vi "ble_search_characteristic_declaration_handle.vi"(8 "error in (no error)":errorcluster, 9 "Characteristic UUID":string, 10 "Service UUID":string, 11 "Handle table":string[][](array[string])) -> (0 "error out":errorcluster, 2 "Handle":string)   [LabVIEW 2013]
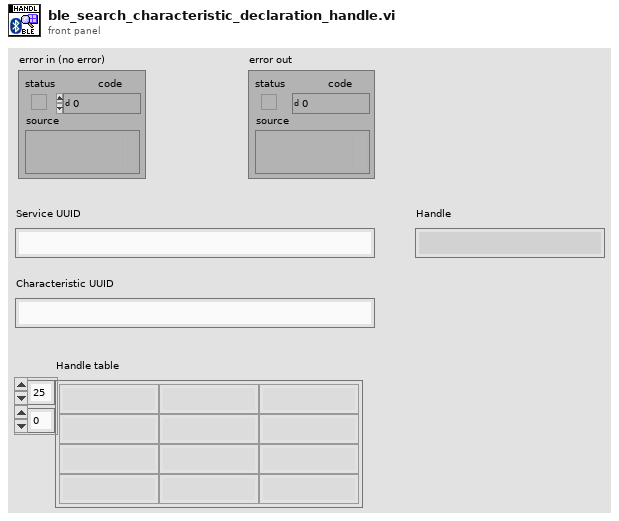
[diagram p1: front panel]
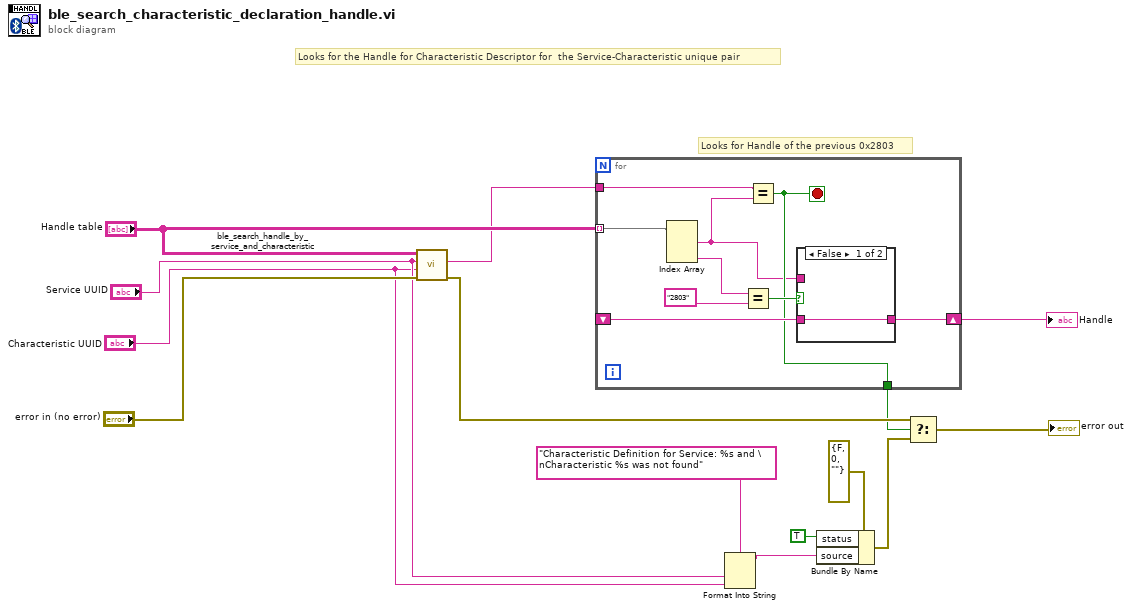
[diagram p0: block diagram]
diagram:
  # "Looks for Handle of the previous 0x2803"
  # "Looks for the Handle for Characteristic Descriptor for  the Service-Characteristic unique pair"
  n1 = call "ble_search_handle_by_service_and_characteristic.vi"("error in (no error)"="error in (no error)", "Characteristic UUID"="Characteristic UUID", "Service UUID"="Service UUID", "Handle table"="Handle table") -> ("error out"=w8:errorcluster, "Handle"=w6:string)  [unwired: 6 in]
  n2 = for {
    tunnel: "Handle table" -> [w23] mode=indexing
    tunnel: w6 -> [w22]
    shift-right: [w19] -> w3
    shift-left: _ -> [w18]
    tunnel: [w17] -> w5
    stop <- w17 stop-if-true
    n3 = Index Array(array=w23) -> (element #1=w16:string, element #3=w15:string)  [unwired: 3 in, 1 out]
    n4 = Equal?(x=w15, y="2803") -> (x = y?=w20:bool)
    n5 = Equal?(x=w22, y=w16) -> (x = y?=w17:bool)
    n6 = case shown="False" w20 {
      tunnel: w16 -> [_ w25]
      tunnel: [w24 w25] -> w19
      tunnel: w18 -> [w24 _]
      frame False {
      }
      frame True {
      }
    }
  }
  "Handle" <- w3
  n7 = Format Into String(format string="Characteristic Definition for Service: %s and \nCharacteristic %s was not found", "Service UUID", "Characteristic UUID") -> (resulting string=w10:string)  [unwired: 2 in, 1 out]
  n8 = Bundle By Name(cluster=errorcluster {"status"=FALSE, "code"=0, "source"=""} ("error in (no error)"), "status"=TRUE, "source"=w10) -> (w13:errorcluster)
  n9 = Select(t=w8, s=w5, f=w13) -> (s? t:f=→"error out":errorcluster)
